vi "NF LI56xx dvr VOLTage psd1 AC RANGe AUTO.vi"(8 "error in":errorcluster caption="error in (no error)" {"code" format="%.0x"}, 9 "Read(F)":bool, 10 "set AC range auto":bool, 11 "VISA resource name":refnum<visa-resource-name>) -> (0 "error out":errorcluster {"code" format="%.0x"}, 2 "query AC range \nauto":bool, 3 "VISA resource name copy":refnum<visa-resource-name>)   [LabVIEW 2019]
doc: "Sets/queries the voltage sensitivity continuous automatic selection function. \nWhen voltage sensitivity is set automatically, dynamic reserve is also set automatically."
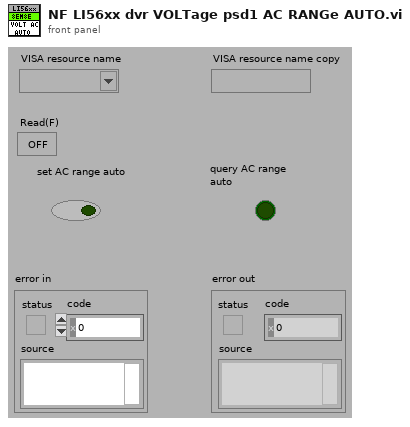
[diagram p1: front panel]
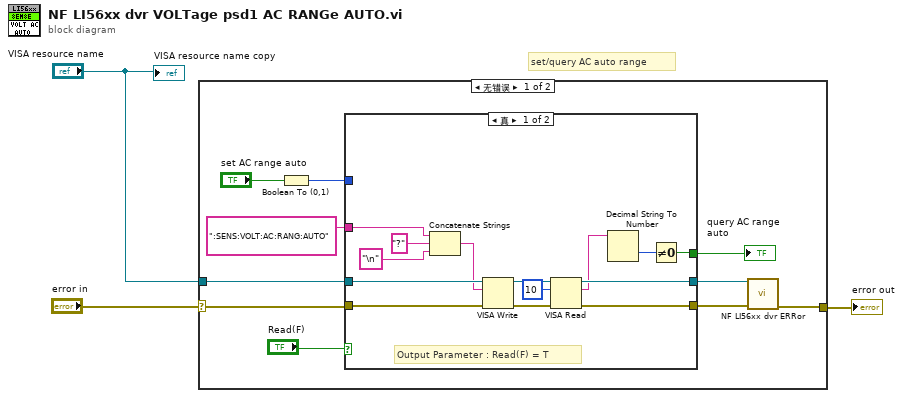
[diagram p0: block diagram]
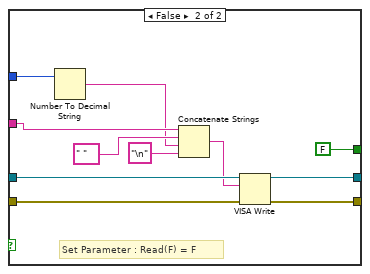
[diagram p2: hidden frame]
diagram:
  # "set/query AC auto range"
  n1 = case shown="无错误" "error in" {
    selector: "error in" -> [w12 w39]
    tunnel: [w8 w39] -> w3
    tunnel: "VISA resource name" -> [w11 _]
    frame No Error {
      n2 = Boolean To (0,1)(Boolean="set AC range auto") -> (0, 1=w6:i16)
      n3 = case shown="真" "Read(F)" {
        tunnel: w11 -> [w27 w38]
        tunnel: [w24 w35] -> w10
        tunnel: [w23 w36] -> w9
        tunnel: w12 -> [w22 w37]
        tunnel: ":SENS:VOLT:AC:RANG:AUTO" ("•¶Žš—ñ") -> [w17 w31]
        tunnel: w6 -> [_ w30]
        tunnel: [w14 FALSE ("query offset enable")] -> w5
        frame True {
          # "Output Parameter : Read(F) = T"
          n4 = Concatenate Strings(w17, "?" ("Œ`Ž®•¶Žš—ñ"), "\n" ("Œ`Ž®•¶Žš—ñ")) -> (w19:string)
          n5 = VISA Write(VISA resource name=w27, write buffer=w19, error in (no error)=w22) -> (VISA resource name out=w25:refnum<visa-resource-name>, error out=w26:errorcluster)  [unwired: 1 out]
          n6 = VISA Read(VISA resource name=w25, byte count=u32 10 ("バイトカウント（0）"), error in (no error)=w26) -> (VISA resource name out=w24:refnum<visa-resource-name>, read buffer=w15:string, error out=w23:errorcluster)  [unwired: 1 out]
          n7 = Decimal String To Number(string=w15) -> (number=w16:i32)  [unwired: 2 in, 1 out]
          n8 = Not Equal To 0?(x=w16) -> (x != 0?=w14:bool)
        }
        frame False {
          # "Set Parameter : Read(F) = F"
          n9 = Number To Decimal String(number=w30) -> (decimal integer string=w29:string)  [unwired: 1 in]
          n10 = Concatenate Strings(w31, " ", w29, "\n" ("Œ`Ž®•¶Žš—ñ")) -> (w34:string)
          n11 = VISA Write(VISA resource name=w38, write buffer=w34, error in (no error)=w37) -> (VISA resource name out=w35:refnum<visa-resource-name>, error out=w36:errorcluster)  [unwired: 1 out]
        }
      }
      "query AC range \nauto" <- w5
      n12 = call "NF LI56xx dvr ERRor.vi"("VISA resource name"=w10, "error in (no error)"=w9) -> ("error out"=w8:errorcluster)  [unwired: 10 in, 3 out]
    }
    frame Error {
    }
  }
  "error out" <- w3
  "VISA resource name copy" <- "VISA resource name"
